vi "SDI-12 Single Operation with output cluster.vi"(0 "RS232 Port In":refnum<visa-resource-name>="COM11", 1 "Sensor Address In":string="0", 4 "Sonde Data Ctl Refnum":refnum<vi>, 7 "Error In (No Error)":errorcluster, 8 "file directory (dialog if empty)":path=path "D:/Cascade/Raw Data files", 9 "Save File":bool, 12 "Time Array In":dbl[](array[numeric]), 13 "Measurement Array In":dbl[][](array[numeric])) -> (14 "time array out":dbl[](array[numeric]), 15 "Measurements Out":dbl[](array[numeric]), 16 "new file path (Not A Path if cancelled)":path, 17 "Time Array":timestamp[](array[timestamp]), 21 "Address Out":string="a" caption="sensor address out", 22 "Measurement  array Out":dbl[][](array[numeric]), 23 "output cluster":T1 caption="Cluster" {"Dissolved\nOxygen (%)" format="%_3g"; "Salinity" format="%_2g"; "Temp (deg C)" format="%_4g"; "ORP" format="%_4g"; "pH" format="%_3g"; "Dissolved\nOxygen mg/L" format="%_4g"; "Specific\nCond (uS)" format="%#_4g"}, 24 "Temperature":cluster{"Y":dbl[], "Y":dbl[]}[](graph), 25 "Sonde Data Display":T2, 27 "Error Out":errorcluster)   [LabVIEW 2016]
doc: "A general set of examples of the SDI-12 API for a generic sensor. A tab control separates each example, and contains the following examples:\n1. Read Single.\n2. Read Multiple.\n3. Acknowledge Active.\n4. Change Address.\n5. Address Query.\n6. Send Identification."
uses:
  SDI-12/Sonde Vertical Graph.ctl
  controls/Vertical Chart.ctl
  activeXtest/activeXtest 2015 Folder/sonde cluster.ctl
  <vilib>/Utility/file.llb/Write Delimited Spreadsheet (string).vi
  SDI-12/SDI-12.lvlib
panel:
  out "loop counter":i32
  out "Error Out 3":errorcluster
  out "error out 2":errorcluster
  out "Error Out 2":errorcluster
  out "error out":errorcluster
  out "Sensor On/Off Response":bool
  out "Battery Voltage (V)":dbl
  out "Number of Measurements Out":i32
  in  "Measurement Type In (Normal)":i32(ring)=1 items=["Normal", "Concurrent", "Continuous"]
  out "Parameter Out":i32(ring) items=["0", "1", "2", "3", "4", "5", "6", "7", "8", "9"]
  in  "Parameter In (0)":i32(ring) items=["0", "1", "2", "3", "4", "5", "6", "7", "8", "9"]
  in  "CRC (False)":bool
  out "CRC Out":bool
  out "Measurement Type Out":i32(ring) items=["Normal", "Concurrent", "Continuous"]
  out "Time (s)":dbl
  out "start time":timestamp
  # "deg C"
  # "pH"
  # "specific conductance mS"
  # "salinity"
  # "DO % saturation"
  # "DO mg/L"
  # "ORP"
  # "depth"
  # "battery"
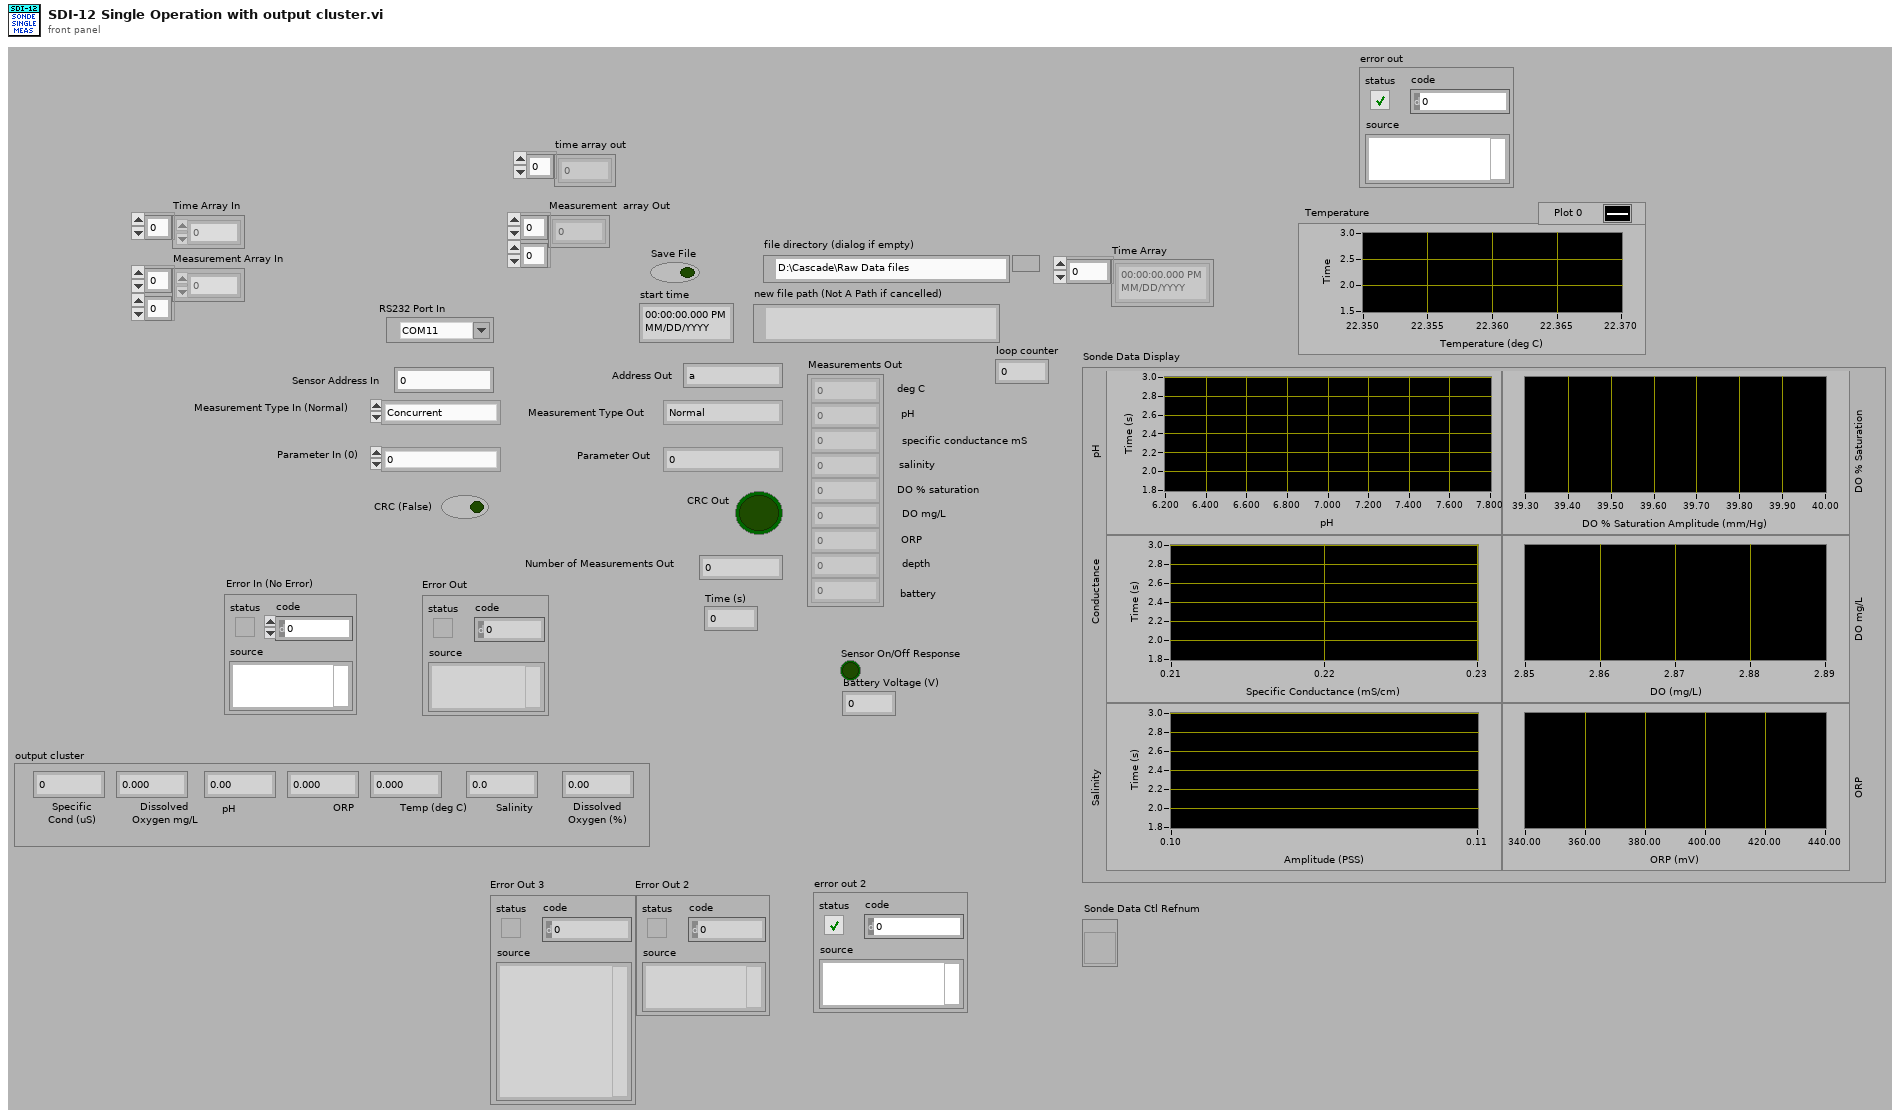
[diagram p1: front panel]
types:
  T1 = typedef "sonde cluster.ctl" = cluster{"Specific\nCond (uS)":dbl, "Dissolved\nOxygen mg/L":dbl, "pH":dbl, "ORP":dbl, "Temp (deg C)":dbl, "Salinity":dbl, "Dissolved\nOxygen (%)":dbl}
  T2 = typedef "Sonde Vertical Graph.ctl" = cluster{"pH":T3, "Conductance":T3, "Salinity":T3, "DO % Saturation":T3, "DO mg/L":T3, "ORP":T3}
  T3 = typedef "Vertical Chart.ctl" = cluster{"Y":dbl[], "Y":dbl[]}[]
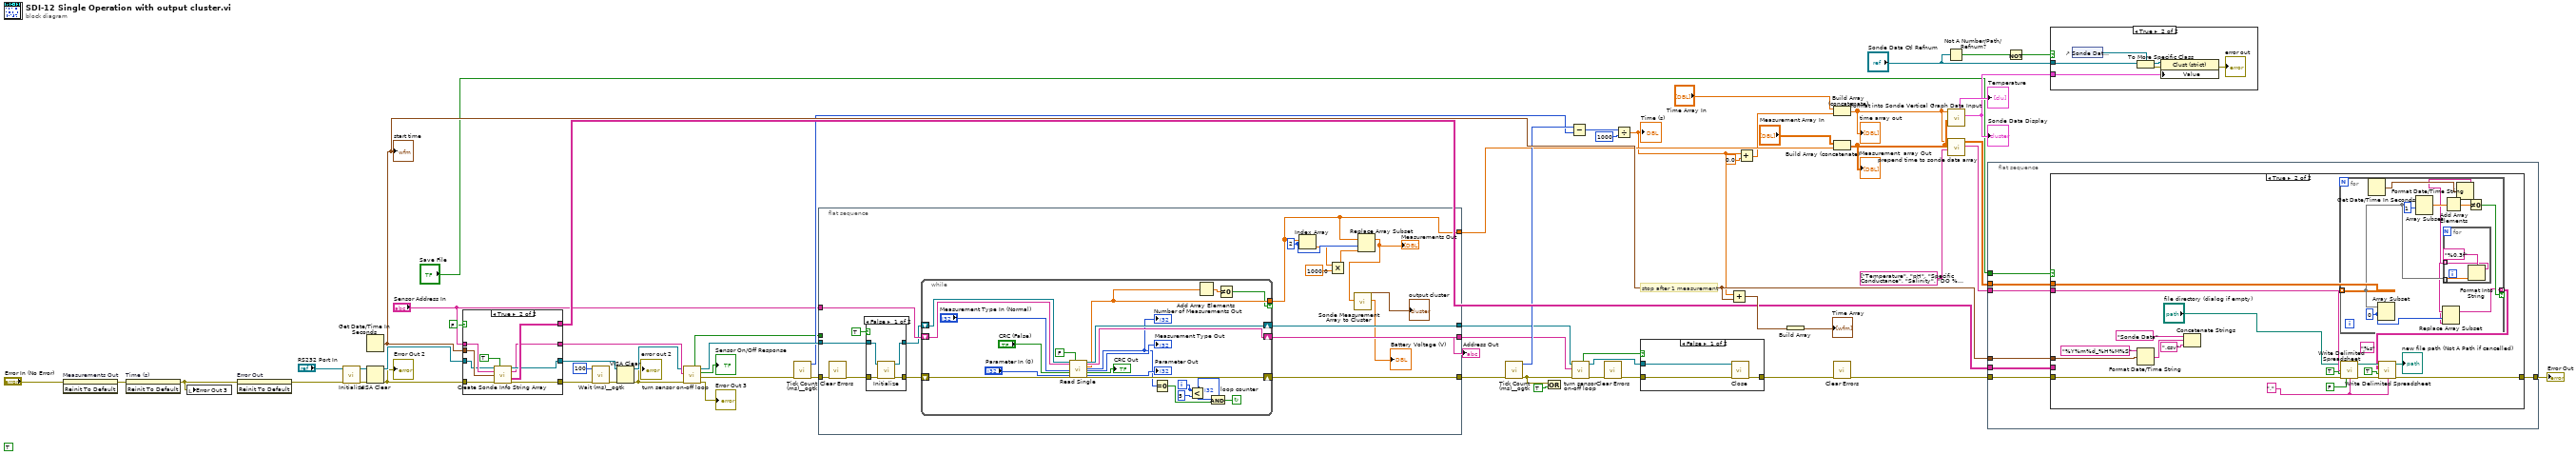
[diagram p0: block diagram]
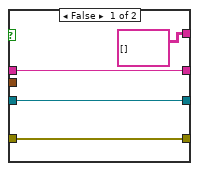
[diagram p2: hidden frame]
diagram:
  (unwired) TRUE ("Sensor On/Off")
  # "stop after 1 measurement"
  n1 = invoke on="Measurements Out" class="Arr (strict)" method="Reinit To Default"(error in="Error In (No Error)") -> (error out=w4:errorcluster)  [unwired: 2 in, 2 out]
  n2 = invoke on="Time (s)" class="DigNum (strict)" method="Reinit To Default"(error in=w4) -> (error out=w2:errorcluster)  [unwired: 2 in, 2 out]
  n3 = local write "Error Out 3"(w2) -> ()
  n4 = invoke on="Error Out" class="Clust (strict)" method="Reinit To Default"(error in=w2) -> (error out=w26:errorcluster)  [unwired: 2 in, 2 out]
  n5 = call "Initialize.vi"("Error In (No Error)"=w26, "RS232 Port In"="RS232 Port In") -> ("Error Out"=w17:errorcluster, "RS232 Port Out"=w60:refnum<visa-resource-name>)  [unwired: 8 in]
  n6 = Get Date/Time In Seconds() -> (seconds since 1Jan1904=w53:timestamp)
  "start time" <- w53
  n7 = VISA Clear(VISA resource name=w60, error in (no error)=w17) -> (VISA resource name out=w18:refnum<visa-resource-name>, error out=w16:errorcluster)
  "Error Out 2" <- w16
  n8 = case shown="True" FALSE {
    tunnel: w53 -> [_ w74]
    tunnel: [string[][] [] ("Array") w73] -> w52
    tunnel: [w64 w72] -> w45
    tunnel: [w63 w71] -> w43
    tunnel: [w65 w70] -> w24
    tunnel: "Sensor Address In" -> [w63 w69]
    tunnel: w18 -> [w64 w68]
    tunnel: w16 -> [w65 w67]
    frame False {
    }
    frame True {
      n9 = call "Create Sonde Info String Array.vi"("VISA Refnum in"=w68, "Initialize/Close?"=TRUE, "Sensor Address In"=w69, "seconds since 1Jan1904"=w74, "error in (no error)"=w67) -> ("VISA Refnum out"=w72:refnum<visa-resource-name>, "Address Out"=w71:string, "Array"=w73:string[][], "error out"=w70:errorcluster)  [unwired: 7 in]
    }
  }
  n10 = call <userlib>:"Wait (ms)__ogtk.vi"("error in (no error)"=w24, "milliseconds to wait"=u32 100) -> ("error out"=w22:errorcluster)  [unwired: 8 in, 1 out]
  n11 = VISA Clear(VISA resource name=w45, error in (no error)=w22) -> (VISA resource name out=w25:refnum<visa-resource-name>, error out=w23:errorcluster)
  "error out 2" <- w23
  n12 = call "turn sensor on-off loop.vi"("error in (no error)"=w23, "Address Out"=w43, "VISA Refnum in"=w25) -> ("error out"=→"Error Out 3":errorcluster, "error out 2"=w46:errorcluster, "Sensor On/Off Response"=→"Sensor On/Off Response":bool, "VISA Refnum out"=w44:refnum<visa-resource-name>, "Initialize/Close?"=w15:bool)  [unwired: 4 in]
  n13 = call <userlib>:"Tick Count (ms)__ogtk.vi"("error in (no error)"=w46) -> ("error out"=w41:errorcluster, "millisecond timer value"=w39:u32)  [unwired: 9 in]
  n14 = flat-sequence {
    tunnel: [w92] -> w12
    tunnel: [w91] -> w42
    tunnel: w41 -> [w90]
    tunnel: w44 -> [w86]
    tunnel: [w81] -> w36
    tunnel: "Sensor Address In" -> [w89]
    tunnel: [w88] -> w9
    tunnel: w15 -> [_]
    frame #0 {
      w80 = 2 ("index")
      n15 = call <vilib>:"Clear Errors.vi"("error in (no error)"=w90) -> ("error out"=w87:errorcluster)  [unwired: 5 in, 1 out]
      n16 = case shown="False" TRUE {
        tunnel: w87 -> [w118 w120]
        tunnel: w86 -> [w117 w119]
        tunnel: [w116 w120] -> w85
        tunnel: [w115 w119] -> w84
        frame False {
          n17 = call "Initialize.vi"("Error In (No Error)"=w118, "RS232 Port In"=w117) -> ("Error Out"=w116:errorcluster, "RS232 Port Out"=w115:refnum<visa-resource-name>)  [unwired: 8 in]
        }
        frame True {
        }
      }
      n18 = while {
        tunnel: [w95] -> w81 if=w93
        shift-right: [w105] -> w88
        shift-left: w89 -> [w106]
        shift-right: [w113] -> w91
        shift-left: w85 -> [w104]
        shift-right: [w114] -> w92
        shift-left: w84 -> [w103]
        i -> [w98]
        stop <- w99 continue-if-true
        n19 = call "Read Single.vi"("RS232 Port In"=w103, "Sensor Address In"=w106, "Measurement Type In (Normal)"="Measurement Type In (Normal)", "CRC (False)"="CRC (False)", "Parameter In (0)"="Parameter In (0)", "Error In (No Error)"=w104, "Initialize/close"=FALSE) -> ("RS232 Port Out"=w114:refnum<visa-resource-name>, "Sensor Address Out"=w105:string, "Measurements Out"=w95:dbl[], "Number of Measurements Out"=w101:i32, "Measurement Type Out"=→"Measurement Type Out":i32, "CRC Out"=→"CRC Out":bool, "Parameter Out"=→"Parameter Out":i32, "Error Out"=w113:errorcluster)  [unwired: 13 in]
        "Number of Measurements Out" <- w101
        n20 = Equal To 0?(x=w101) -> (x = 0?=w100:bool)
        n21 = Less?(x=w98, y=5) -> (x < y?=w96:bool)
        n22 = Add Array Elements(numeric array=w95) -> (sum=w94:dbl)
        n23 = And(x=w96, y=w100) -> (x .and. y?=w99:bool)
        n24 = Not Equal To 0?(x=w94) -> (x != 0?=w93:bool)
        "loop counter" <- w98
      }
      n25 = Index Array(array=w81, index=w80) -> (element=w79:dbl)
      n26 = Multiply(x=w79, y=1000.0) -> (x*y=w78:dbl)
      n27 = Replace Array Subset(array=w81, new element=w78, index=w80) -> (w75:dbl[])
      "Measurements Out" <- w75
      n28 = call "Sonde Measurement Array to Cluster.vi"("Measurements In"=w75) -> ("Battery Voltage (V)"=→"Battery Voltage (V)":dbl, "Cluster Out"=→"output cluster":T1)  [unwired: 9 in]
    }
  }
  n29 = call <userlib>:"Tick Count (ms)__ogtk.vi"("error in (no error)"=w42) -> ("error out"=w11:errorcluster, "millisecond timer value"=w40:u32)  [unwired: 9 in]
  n30 = Compound Arithmetic op=OR(w11, TRUE) -> ()  [unwired: 1 out]
  n31 = Subtract(x=w40, y=w39) -> (x-y=w38:u32)
  n32 = call "turn sensor on-off loop.vi"("error in (no error)"=w11, "Address Out"=w9, "VISA Refnum in"=w12) -> ("error out"=w8:errorcluster, "VISA Refnum out"=w10:refnum<visa-resource-name>, "Initialize/Close?"=w7:bool)  [unwired: 4 in, 2 out]
  n33 = call <vilib>:"Clear Errors.vi"("error in (no error)"=w8) -> ("error out"=w19:errorcluster)  [unwired: 5 in, 1 out]
  n34 = Divide(x=w38, y=u32 1000) -> (x/y=w35:dbl)
  "Time (s)" <- w35
  n35 = case shown="False" w7 {
    tunnel: [w123 w124] -> w56
    tunnel: w19 -> [w122 w124]
    tunnel: w10 -> [w121 _]
    frame False {
      n36 = call "Close.vi"("Error In (No Error)"=w122, "RS232 Port In"=w121) -> ("Error Out"=w123:errorcluster)  [unwired: 9 in]
    }
    frame True {
    }
  }
  n37 = Add(x=w35, y=w53) -> (x+y=w58:timestamp)
  n38 = Add(x=w35, y=0.0) -> (x+y=w34:dbl)
  n39 = Build Array(w58) -> (→"Time Array":timestamp[])
  n40 = Build Array (concatenate)("Time Array In", w34) -> (w49:dbl[])
  "time array out" <- w49
  n41 = Build Array (concatenate)("Measurement Array In", w36) -> (w57:dbl[][])
  "Measurement  array Out" <- w57
  n42 = call <vilib>:"Clear Errors.vi"("error in (no error)"=w56) -> ("error out"=w6:errorcluster)  [unwired: 5 in, 1 out]
  n43 = Not A Number/Path/Refnum?(number/path/refnum="Sonde Data Ctl Refnum") -> (NaN/Path/Refnum?=w32:bool)
  n44 = call "format into Sonde Vertical Graph Data Input.vi"("Sonde Measurement Array"=w57, "Time Array"=w49) -> ("Sonde Data Display"=w30:T2, "Temperature"=→"Temperature":cluster{"X":dbl[], "Y":dbl[]}[])  [unwired: 8 in]
  "Sonde Data Display" <- w30
  n45 = call "prepend time to sonde data array.vi"("Measurement Labels"=string[] ["Temperature", "pH", "Specific Conductance", "Salinity", "DO % saturation", "DO", "ORP", "depth", "battery"], "Sonde\nData Array"=w57, "Time Array"=w49) -> ("Header Array"=w51:string[], "Data Array"=w54:dbl[][])  [unwired: 7 in]
  n46 = flat-sequence {
    tunnel: w6 -> [w131]
    tunnel: [w130] -> w55
    tunnel: w51 -> [w129]
    tunnel: w54 -> [w128]
    tunnel: w53 -> [w127]
    tunnel: w52 -> [w126]
    tunnel: "Save File" -> [w125]
    frame #0 {
      n47 = case shown="True" w125 {
        tunnel: [w132 w148] -> w130
        tunnel: w131 -> [w132 w136]
        tunnel: w129 -> [_ w137]
        tunnel: w128 -> [_ w134]
        tunnel: w127 -> [_ w142]
        tunnel: w126 -> [_ _]
        frame False {
        }
        frame True {
          (unwired) "%s" ("format (%.3f)")
          w138 = "," ("delimiter (\\t)")
          n48 = Format Date/Time String(time format string (%c)="%Y%m%d_%H%M%S", seconds (now)=w142) -> (date/time string=w141:string)  [unwired: 1 in]
          n49 = Concatenate Strings("Sonde Data" ("name or relative path"), w141, ".csv" ("string")) -> ()  [unwired: 1 out]
          n50 = for {
            tunnel: w134 -> [w154] mode=indexing
            tunnel: [w155] -> w133 mode=indexing if=w159
            w156 = 0 ("index")
            n51 = Get Date/Time In Seconds() -> (seconds since 1Jan1904=w152:timestamp)
            n52 = Array Subset(array=w154, index=w156) -> ()  [unwired: 1 in, 1 out]
            n53 = Array Subset(array=w154, index=1) -> (w158:dbl[])  [unwired: 1 in]
            n54 = for {
              tunnel: w154 -> [w163] mode=indexing
              tunnel: [w161] -> w153 mode=indexing
              n55 = Format Into String(format string="%0.3f", w163) -> (resulting string=w161:string)  [unwired: 2 in, 1 out]
            }
            n56 = Add Array Elements(numeric array=w158) -> (sum=w160:dbl)
            n57 = Format Date/Time String(seconds (now)=w152) -> (date/time string=w151:string)  [unwired: 2 in]
            n58 = Replace Array Subset(array=w153, new element=w151, index=w156) -> (w155:string[])
            n59 = Not Equal To 0?(x=w160) -> (x != 0?=w159:bool)
          }
          n60 = call-poly <vilib>:"Write Delimited Spreadsheet.vi"("file path (dialog if empty)"="file directory (dialog if empty)", "1D data"=w137, "append to file? (new file:F)"=TRUE ("append to file? (F)"), "error in (no error)"=w136, "transpose? (no:F)"=FALSE ("transpose? (F)"), "delimiter (\\t)"=w138) -> ("new file path (Not A Path if cancelled)"=w150:path, "error out"=w149:errorcluster)  [unwired: 8 in]
          n61 = call-poly <vilib>:"Write Delimited Spreadsheet.vi"("file path (dialog if empty)"=w150, "2D data"=w133, "append to file? (new file:F)"=TRUE ("append to file? (F)"), "error in (no error)"=w149, "delimiter (\\t)"=w138) -> ("new file path (Not A Path if cancelled)"=→"new file path (Not A Path if cancelled)":path, "error out"=w148:errorcluster)  [unwired: 9 in]
        }
      }
    }
  }
  n62 = Not(x=w32) -> (.not. x?=w31:bool)
  n63 = case shown="True" w31 {
    tunnel: w30 -> [_ w169]
    tunnel: "Sonde Data Ctl Refnum" -> [_ w167]
    frame False {
    }
    frame True {
      n64 = control-ref of="Sonde Data Display"() -> (w168:refnum<vi>)
      n65 = To More Specific Class(target class=w168, reference=w167) -> (specific class reference=w166:refnum<vi>, error out=w165:errorcluster)  [unwired: 1 in]
      n66 = property class="Clust (strict)"(reference=w166, error in=w165, "Value"=w169) -> (error out=→"error out":errorcluster)  [unwired: 1 out]
    }
  }
  "Error Out" <- w55
  "Address Out" <- w9
